vi "FlowControlTests.vi"() -> ()   [LabVIEW 2016]
panel:
  out "display number":dbl
  out "constant":dbl
  out "other number":u32
  out "text":string
  out "Moving Avg RMS":dbl(slide) scale=0.008..0.02
  in  "Extension":string="_EMG.txt"
  in  "File Name":string
  in  "Data Directory":path=path "C:/Users/Tinggroup/Desktop/VRMuscleActivationVisualizer/LabviewFiles/Jake DCScode_GT/BiofeedbackEMGPackage/EMGData"
  in  "End Trial":bool
  in  "Start Trial":bool
  in  "Frames Per Second":dbl=30.0
  in  "UI Data Input File":path=path "C:/Users/Tinggroup/Desktop/VRMuscleActivationVisualizer/StationaryVisualFeedbackVR/assets/BiofeedbackData.txt"
  in  "Execut Case":bool
  out "second loop":dbl
  in  "Stop Second Loop":bool
  in  "Stop  Big Loop":bool
  out "big loops":dbl
  out "small loops":dbl
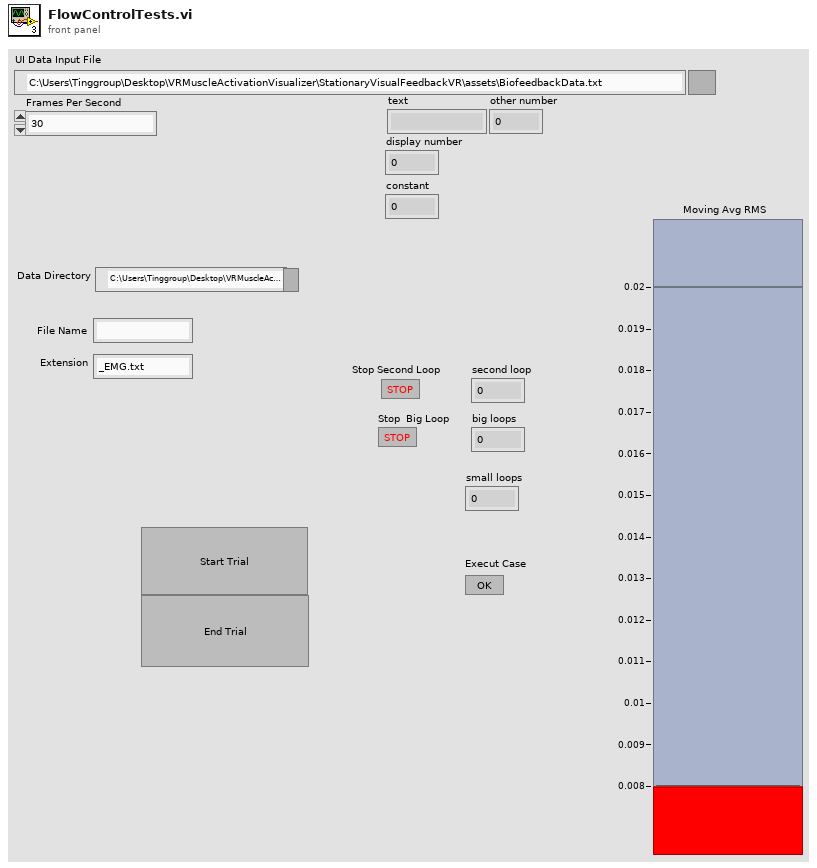
[diagram p1: front panel]
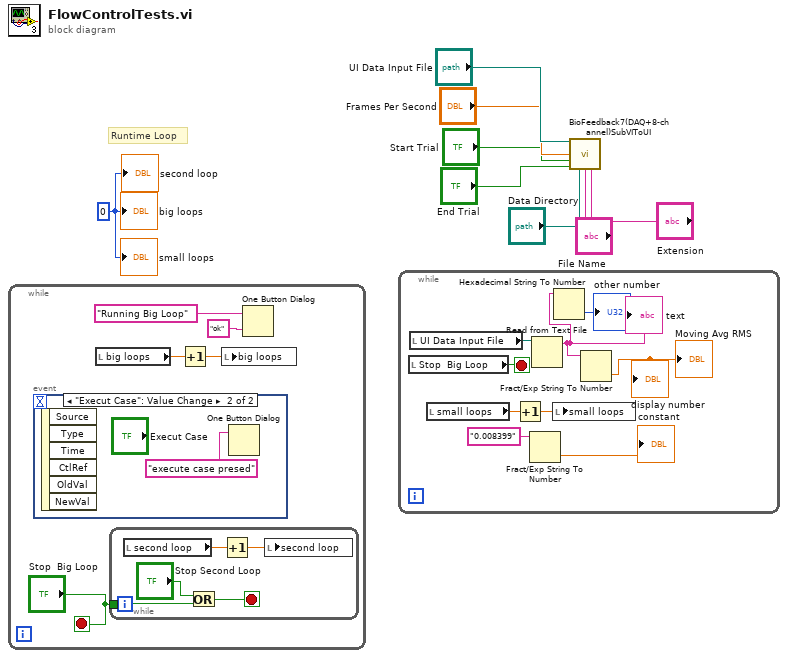
[diagram p0: block diagram]
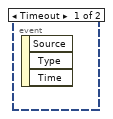
[diagram p2: hidden frame]
diagram:
  w8 = 0
  # "Runtime Loop"
  n1 = while {
    stop <- "Stop  Big Loop" stop-if-true
    n2 = event shown="[1] \"Execut Case\": Value Change" {
      selector: _ -> [_ _]
      dyn-events: _ -> [_ _]
      timeout: _ -> [_ _]
      event Timeout {
        n3 = event-data() -> ()  [unwired: 1 in, 3 out]
      }
      event "Execut Case": Value Change {
        n4 = event-data() -> ()  [unwired: 1 in, 6 out]
        n5 = One Button Dialog(message="execute case presed") -> ()  [unwired: 1 in, 1 out]
      }
    }
    n6 = local read "big loops"() -> (w13:dbl)
    n7 = while {
      tunnel: "Stop  Big Loop" -> [w16]
      stop <- w15 stop-if-true
      n8 = local read "second loop"() -> (w19:dbl)
      n9 = Or(x="Stop Second Loop", y=w16) -> (x .or. y?=w15:bool)
      n10 = Increment(x=w19) -> (x+1=w18:dbl)
      n11 = local write "second loop"(w18) -> ()
    }
    n12 = Increment(x=w13) -> (x+1=w12:dbl)
    n13 = local write "big loops"(w12) -> ()
    n14 = One Button Dialog(message="Running Big Loop", button name ("OK")="ok") -> ()  [unwired: 1 out]
  }
  n15 = while {
    stop <- w27 stop-if-true
    n16 = local read "Stop  Big Loop"() -> (w27:bool)
    n17 = local read "UI Data Input File"() -> (w28:path)
    n18 = local read "small loops"() -> (w25:dbl)
    n19 = Increment(x=w25) -> (x+1=w26:dbl)
    n20 = Fract/Exp String To Number(string="0.008399") -> (number=→"constant":dbl)  [unwired: 3 in, 1 out]
    n21 = Read from Text File(file (use dialog)=w28) -> (text=w21:string)  [unwired: 3 in, 3 out]
    "text" <- w21
    n22 = local write "small loops"(w26) -> ()
    n23 = Hexadecimal String To Number(string=w21) -> (number=→"other number":u32)  [unwired: 2 in, 1 out]
    n24 = Fract/Exp String To Number(string=w21) -> (number=→"Moving Avg RMS" →"display number":dbl)  [unwired: 3 in, 1 out]
  }
  n25 = call "BioFeedback7(DAQ+8-channel)SubVIToUI.vi"("UI Data Input File"="UI Data Input File", "Frames Per Second"="Frames Per Second", "Start Trial"="Start Trial", "End Trial"="End Trial", "Data Directory"="Data Directory", "File Name"="File Name", "Extension"="Extension") -> ()  [unwired: 9 in]
  "small loops" <- w8
  "big loops" <- w8
  "second loop" <- w8
